vi "SDCP BTR Read Parameter File.vi"(2 "error in (no error)":errorcluster, 3 "BTP File Path":path) -> (0 "error out":errorcluster, 1 "BTR parameters":T1[](array[typedef]))   [LabVIEW 2020]
uses:
  Typedefs/SDCP BTR Parameter cluster.ctl
  Typedefs/SDCP BTR Parameter data type.ctl
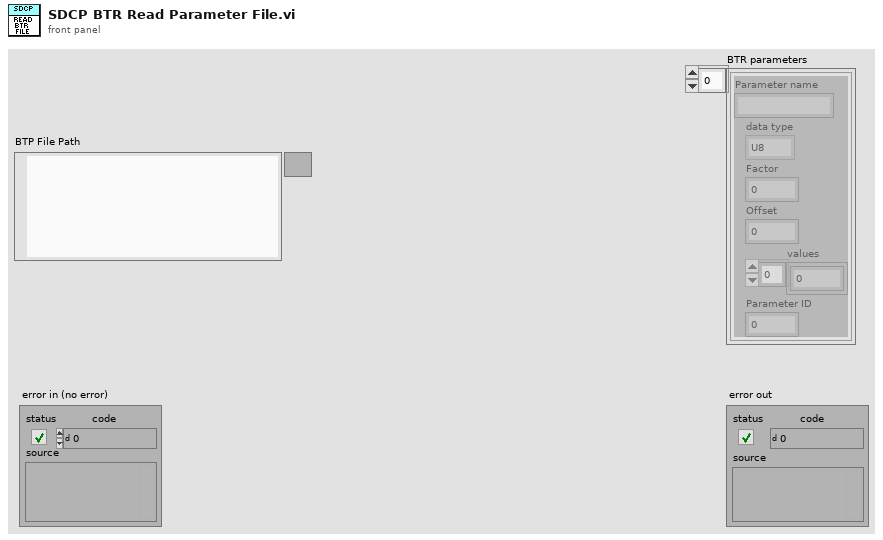
[diagram p1: front panel]
types:
  T1 = typedef "SDCP BTR Parameter cluster.ctl" = cluster{"Parameter name":string, "data type":T2, "Factor":dbl, "Offset":dbl, "values":dbl[], "Parameter ID":i32}
  T2 = typedef "SDCP BTR Parameter data type.ctl" = enum16{"U8", "I8", "U16", "I16", "U32", "I32", "F32"}
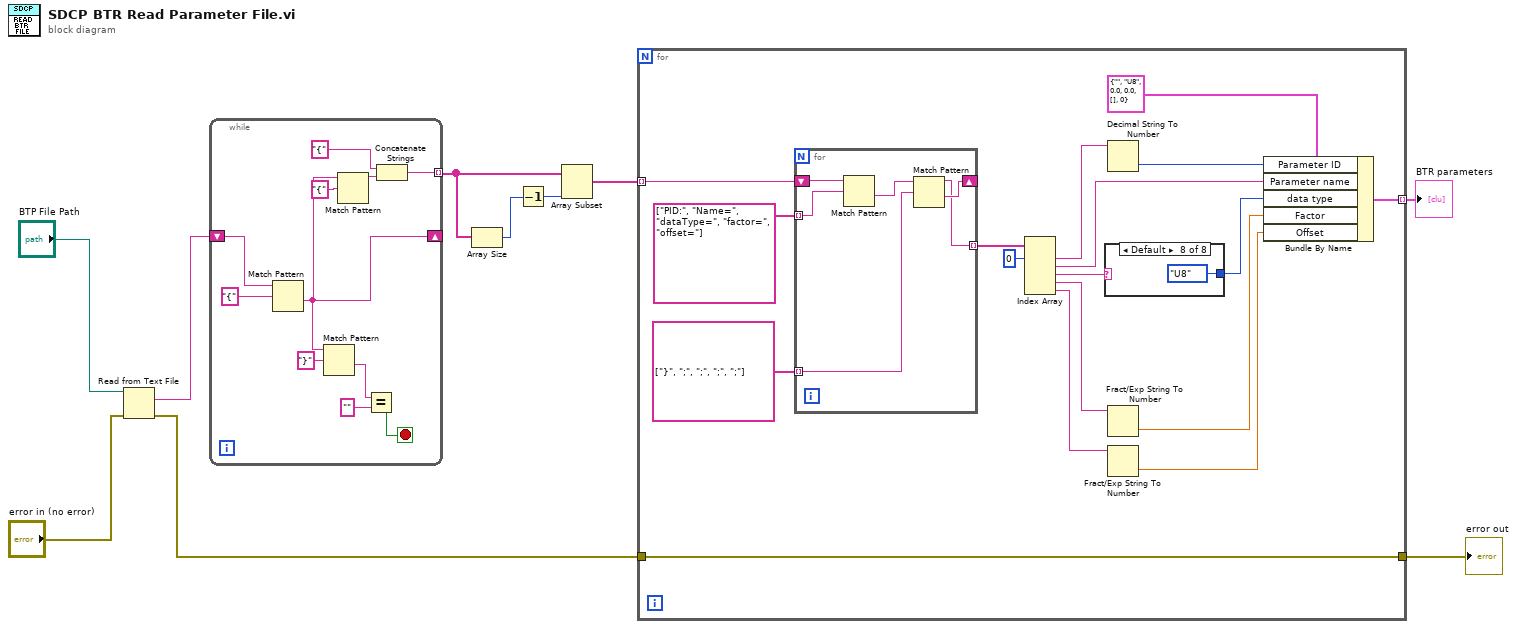
[diagram p0: block diagram]
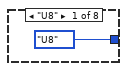
[diagram p2: hidden frame]
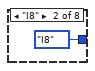
[diagram p3: hidden frame]
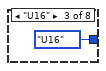
[diagram p4: hidden frame]
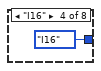
[diagram p5: hidden frame]
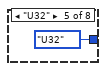
[diagram p6: hidden frame]
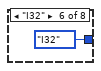
[diagram p7: hidden frame]
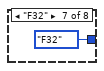
[diagram p8: hidden frame]
diagram:
  n1 = Read from Text File(file (use dialog)="BTP File Path", error in="error in (no error)") -> (text=w8:string, error out=w3:errorcluster)  [unwired: 2 in, 2 out]
  n2 = while {
    shift-right: [w15] -> _
    shift-left: w8 -> [w21]
    tunnel: [w17] -> w7 mode=indexing
    stop <- w13 stop-if-true
    n3 = Match Pattern(string=w21, regular expression="{") -> (after substring=w15:string)  [unwired: 1 in, 3 out]
    n4 = Match Pattern(string=w15, regular expression="}") -> (after substring=w12:string)  [unwired: 1 in, 3 out]
    n5 = Match Pattern(string=w15, regular expression="{") -> (before substring=w18:string)  [unwired: 1 in, 3 out]
    n6 = Equal?(x=w12, y="") -> (x = y?=w13:bool)
    n7 = Concatenate Strings("{" ("string"), w18) -> (w17:string)
  }
  n8 = Array Size(array=w7) -> (size(s)=w5:i32)
  n9 = Decrement(x=w5) -> (x-1=w6:i32)
  n10 = Array Subset(array=w7, length=w6) -> (w4:string[])  [unwired: 1 in]
  n11 = for {
    tunnel: w4 -> [w38] mode=indexing
    tunnel: [w23] -> w1 mode=indexing
    tunnel: w3 -> [w22]
    tunnel: [w22] -> w2
    n12 = for {
      shift-right: [w48] -> _
      shift-left: w38 -> [w52]
      tunnel: string[] ["PID:", "Name=", "dataType=", "factor=", "offset="] -> [w51] mode=indexing
      tunnel: string[] ["}", ";", ";", ";", ";"] -> [w49] mode=indexing
      tunnel: [w47] -> w35 mode=indexing
      n13 = Match Pattern(string=w52, regular expression=w51) -> (after substring=w50:string)  [unwired: 1 in, 3 out]
      n14 = Match Pattern(string=w50, regular expression=w49) -> (before substring=w47:string, after substring=w48:string)  [unwired: 1 in, 2 out]
    }
    n15 = Index Array(array=w35, index #1=0 ("index")) -> (element #1=w33:string, element #2=w27:string, element #3=w30:string, element #4=w32:string, element #5=w31:string)  [unwired: 4 in]
    n16 = case shown="Default" w30 {
      tunnel: [SDCP_BTR_Parameter_data_type."U8" ("Enum") SDCP_BTR_Parameter_data_type."I8" ("Enum") SDCP_BTR_Parameter_data_type."U16" ("Enum") SDCP_BTR_Parameter_data_type."I16" ("Enum") SDCP_BTR_Parameter_data_type."U32" ("Enum") SDCP_BTR_Parameter_data_type."I32" ("Enum") SDCP_BTR_Parameter_data_type."F32" ("Enum") SDCP_BTR_Parameter_data_type."U8" ("Enum")] -> w26
      frame "U8" {
      }
      frame "I8" {
      }
      frame "U16" {
      }
      frame "I16" {
      }
      frame "U32" {
      }
      frame "I32" {
      }
      frame "F32" {
      }
      frame Default {
      }
    }
    n17 = Decimal String To Number(string=w33) -> (number=w28:i32)  [unwired: 2 in, 1 out]
    n18 = Fract/Exp String To Number(string=w32) -> (number=w25:dbl)  [unwired: 3 in, 1 out]
    n19 = Fract/Exp String To Number(string=w31) -> (number=w24:dbl)  [unwired: 3 in, 1 out]
    n20 = Bundle By Name(cluster=T1 {"Parameter name"="", "data type"=enum."U8", "Factor"=0.0, "Offset"=0.0, "values"=[], "Parameter ID"=0}, "Parameter ID"=w28, "Parameter name"=w27, "data type"=w26, "Factor"=w25, "Offset"=w24) -> (w23:T1)
  }
  "error out" <- w2
  "BTR parameters" <- w1
